vi "Write Strr.vi"(8 "error in (no error)":errorcluster, 10 "Strr":string, 11 "In":refnum<class "class1.lvclass">) -> (0 "error out":errorcluster, 3 "Out":refnum<class "class1.lvclass">)   [LabVIEW 2018, in "class1.lvclass"]
uses:
  class1.lvclass
  class1.lvclass/class1.ctl
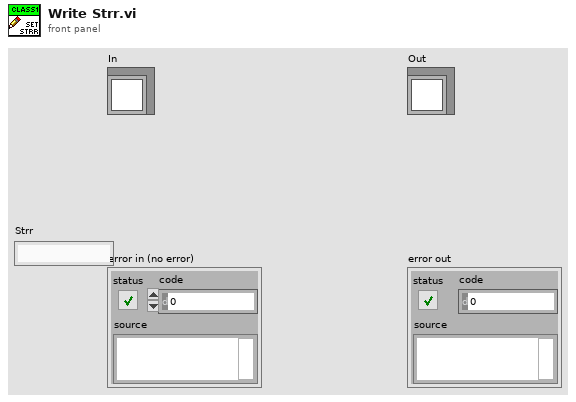
[diagram p1: front panel]
types:
  T1 = typedef "class1.lvclass/Data.ctl" = cluster{"Path":path, "ID":string, "Settings":T2, "asdf":enum16{"a", "f"}, "XY Graph":cluster{"X":dbl, "Y":dbl}[]}
  T2 = typedef "class1.lvclass/Settings.ctl" = cluster{"Speed":dbl, "Strr":string, "data":i32[]}
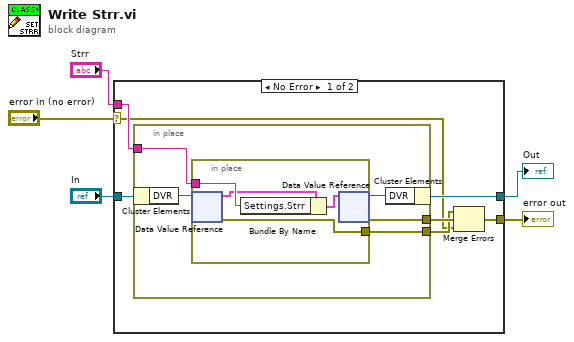
[diagram p0: block diagram]
diagram:
  n1 = case shown="No Error" "error in (no error)" {
    selector: "error in (no error)" -> [w6 w23]
    tunnel: [w7 w23] -> w4
    tunnel: [w12 w22] -> w3
    tunnel: "In" -> [w11 w22]
    tunnel: "Strr" -> [w10 _]
    frame No Error {
      n2 = in-place {
        in-place-border: w10 -> [w15]
        in-place-border: [w14] -> w9
        in-place-border: [w13] -> w8
        n3 = in-place-cluster #1(w11) -> ("DVR"=w16:refnum<data-value>)
        n4 = in-place {
          in-place-border: w15 -> [w20]
          in-place-border: [w18] -> w13
          n5 = in-place-dvr #2(w16) -> (w19:T1, w18:errorcluster)
          n6 = Bundle By Name(cluster=w19, "Settings.Strr"=w20) -> (w21:T1)
          n7 = in-place-dvr #2(w21) -> (w17:refnum<data-value>, w14:errorcluster)
        }
        n8 = in-place-cluster #1("DVR"=w17) -> (w12:refnum<class "class1.lvclass">)
      }
      n9 = Merge Errors(w8, w9, w6) -> (w7:errorcluster)
    }
    frame Error {
    }
  }
  "Out" <- w3
  "error out" <- w4
